vi "Send UI Message.vi"(8 "error in (no error)":errorcluster, 9 "Data":variant, 10 "Msg":T1, 11 "UI Queue":refnum<queue>) -> (0 "error out":errorcluster)   [LabVIEW 2015, in "Execution.lvclass"]
uses:
  Execution.lvclass
  EXECUTION_UI_MSG.ctl
  EXECUTION_UI_QUEUE_DATA.ctl
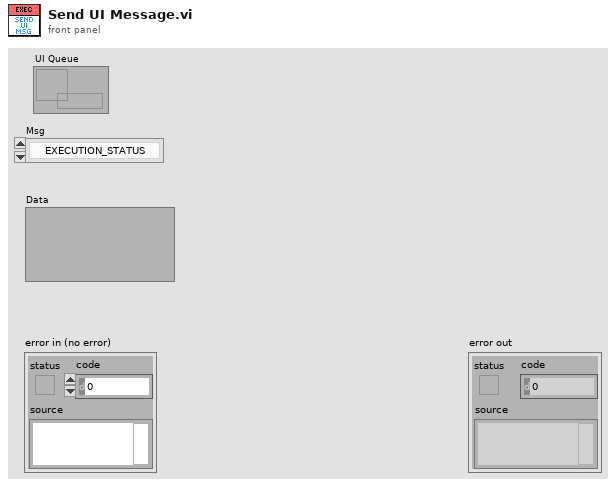
[diagram p1: front panel]
types:
  T1 = typedef "Execution.lvclass/EXECUTION_UI_MSG.ctl" = enum16{"EXECUTION_STATUS", "INIT_UI", "DUT_UPDATE", "BOTTOM_PANEL_UPDATE", "TOP_PANEL_UPDATE", "STEP_START", "STEP_END", "DISPLAY_RESULT", "APPLICATION_END"}
  T2 = typedef "Execution.lvclass/EXECUTION_UI_QUEUE_DATA.ctl" = cluster{"Msg":T1, "Data":variant}
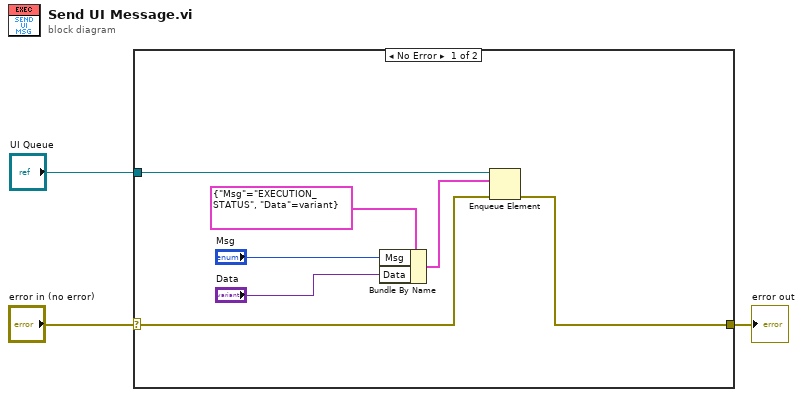
[diagram p0: block diagram]
diagram:
  n1 = case shown="No Error" "error in (no error)" {
    selector: "error in (no error)" -> [w6 w11]
    tunnel: [w5 w11] -> w2
    tunnel: "UI Queue" -> [w4 _]
    frame No Error {
      n2 = Bundle By Name(cluster=T2 {"Msg"=enum."EXECUTION_STATUS", "Data"=variant} ("element"), "Msg"="Msg", "Data"="Data") -> (w9:T2)
      n3 = Enqueue Element(queue=w4, element=w9, error in (no error)=w6) -> (error out=w5:errorcluster)  [unwired: 1 in, 2 out]
    }
    frame Error {
    }
  }
  "error out" <- w2
